vi "Area.vi"(8 "error in (no error)":errorcluster, 11 "Line in":refnum<class "Line.lvclass">) -> (0 "error out":errorcluster, 2 "rect":T1, 3 "Line out":refnum<class "Line.lvclass">)   [LabVIEW 2021, in "Picture2D.lvlib" / "Line.lvclass"]
uses:
  Line.lvclass
  Shape/Shape.lvclass
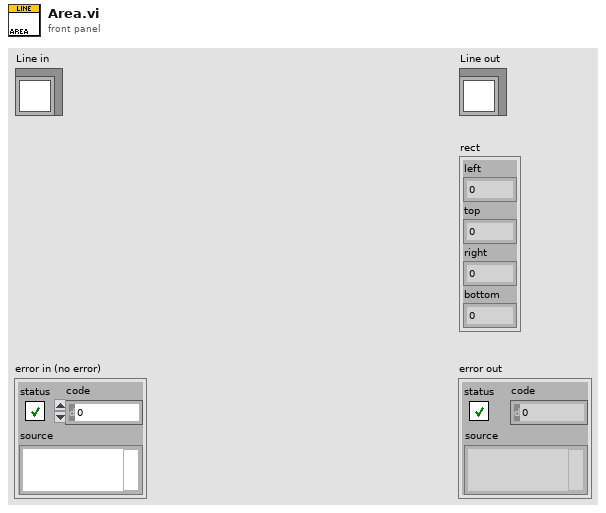
[diagram p1: front panel]
types:
  T1 = cluster{"left":i16, "top":i16, "right":i16, "bottom":i16}
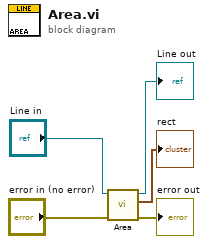
[diagram p0: block diagram]
diagram:
  n1 = call-parent "Area.vi"("error in (no error)"="error in (no error)", "Shape in"="Line in") -> ("error out"=→"error out":errorcluster, "rect"=→"rect":T1, "Shape out"=→"Line out":refnum<class "Line.lvclass">)  [unwired: 7 in]
